vi "UserProgramNewtonSolver.vi"() -> ()   [LabVIEW 2021]
panel:
  out "Root":dbl
  in  "stop":bool
  in  "Rootfinder":T1
  # "x²+"
  # "x"
  # "+"
  # "=0"
  # "Coefficients:"
  # "Initial condition:"
  # "Bounds:"
  # "<x<"
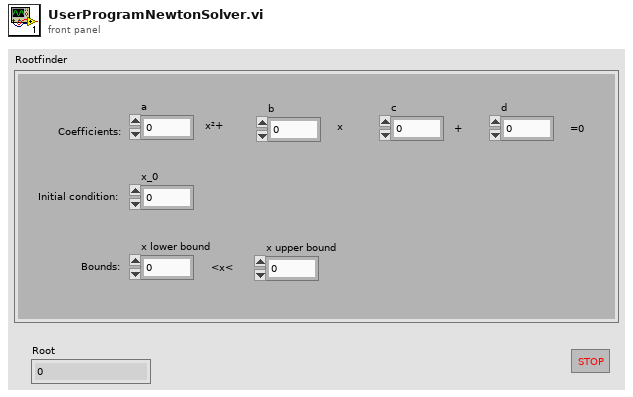
[diagram p1: front panel]
types:
  T1 = cluster{"a":dbl, "b":dbl, "c":dbl, "x_0":dbl, "x lower bound":dbl, "x upper bound":dbl, "d":dbl}
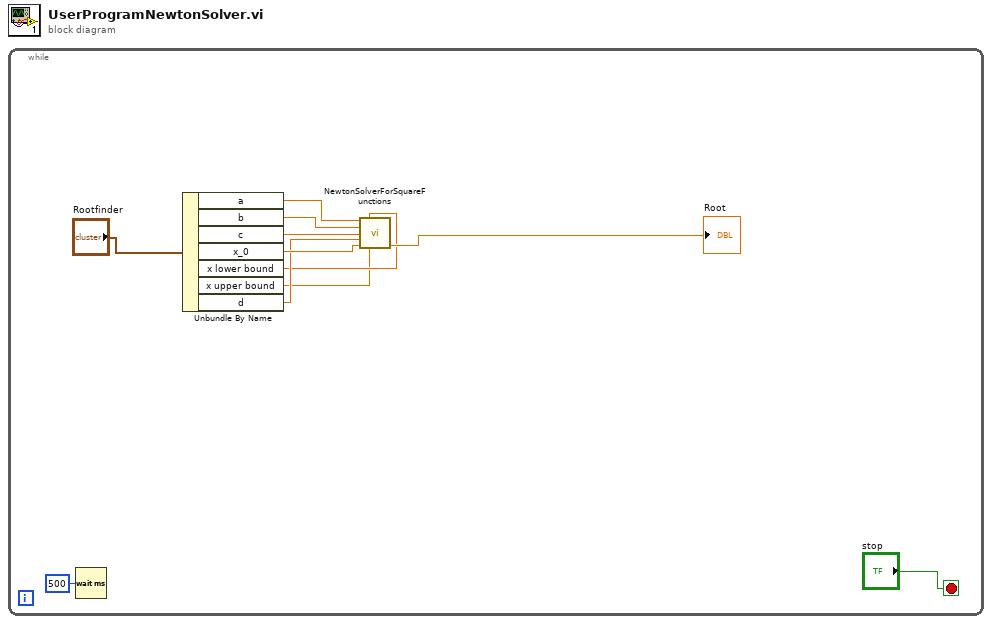
[diagram p0: block diagram]
diagram:
  n1 = while {
    stop <- "stop" stop-if-true
    n2 = Wait (ms)(milliseconds to wait=u32 500 ("millisecond timer value")) -> ()  [unwired: 1 out]
    n3 = Unbundle By Name("Rootfinder") -> ("a"=w7:dbl, "b"=w6:dbl, "c"=w5:dbl, "x_0"=w4:dbl, "x lower bound"=w2:dbl, "x upper bound"=w1:dbl, "d"=w3:dbl)
    n4 = call "NewtonSolverForSquareFunctions.vi"("a"=w7, "x lower bound"=w2, "b"=w6, "c"=w5, "d"=w3, "x_0"=w4, "x upper bound"=w1) -> ("x_n"=→"Root":dbl)  [unwired: 8 in]
  }
